vi "caculate actual pos.vi"(6 "robot org y":dbl=4.0, 7 "robot org x":dbl=2.0, 9 "camera y":dbl=8.0, 10 "camera x":dbl=5.0, 11 "Array":dbl[](array[numeric])) -> (2 "robot y":dbl, 3 "robot x":dbl)   [LabVIEW 2016]
panel:
  out "appended array":dbl[][](array[numeric])
  out "Array 2":dbl[](array[numeric])
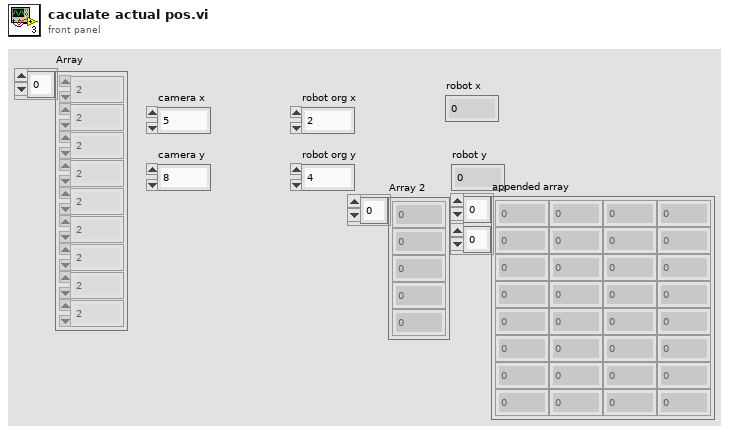
[diagram p1: front panel]
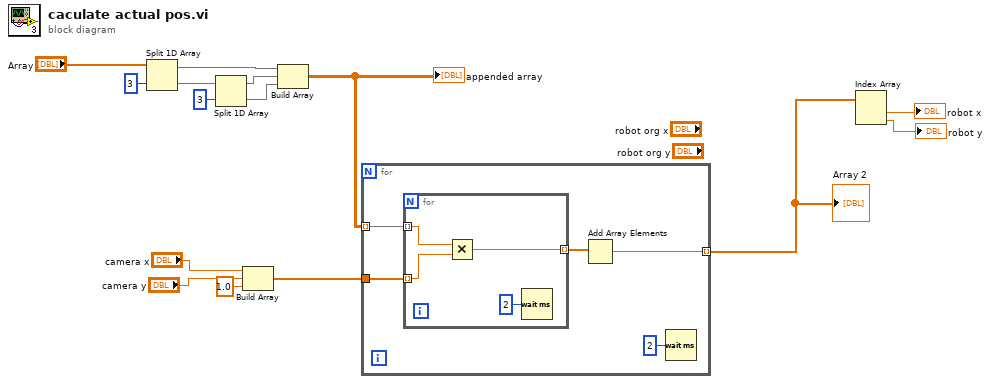
[diagram p0: block diagram]
diagram:
  n1 = Split 1D Array(array="Array", index=3) -> (first subarray=w12:dbl[], second subarray=w13:dbl[])
  n2 = Split 1D Array(array=w13, index=3) -> (first subarray=w11:dbl[], second subarray=w10:dbl[])
  n3 = Build Array("camera x", "camera y", 1.0 ("element")) -> (w3:dbl[])
  n4 = Build Array "Build Array"(w12, w11, w10) -> (w4:dbl[][])
  "appended array" <- w4
  n5 = for {
    tunnel: w4 -> [w20] mode=indexing
    tunnel: w3 -> [w19]
    tunnel: [w17] -> w1 mode=indexing
    n6 = for {
      tunnel: w20 -> [w23] mode=indexing
      tunnel: w19 -> [w22] mode=indexing
      tunnel: [w24] -> w18 mode=indexing
      n7 = Multiply(x=w23, y=w22) -> (x*y=w24:dbl)
      n8 = Wait (ms)(milliseconds to wait=u32 2 ("等待时间（毫秒）")) -> ()  [unwired: 1 out]
    }
    n9 = Add Array Elements(numeric array=w18) -> (sum=w17:dbl)
    n10 = Wait (ms)(milliseconds to wait=u32 2 ("等待时间（毫秒）")) -> ()  [unwired: 1 out]
  }
  "Array 2" <- w1
  n11 = Index Array "Index Array"(array=w1) -> (element #1=→"robot x":dbl, element #2=→"robot y":dbl)  [unwired: 2 in]
